vi "Read and Write type1.vi"(8 "error in":errorcluster, 9 "IN":T1(array[cluster]), 10 "Enum":enum16{"Init", "Read", "Write"}(ring), 11 "Path Out":path) -> (0 "error out":errorcluster, 1 "OUT":T1(array[cluster]))   [LabVIEW 2018]
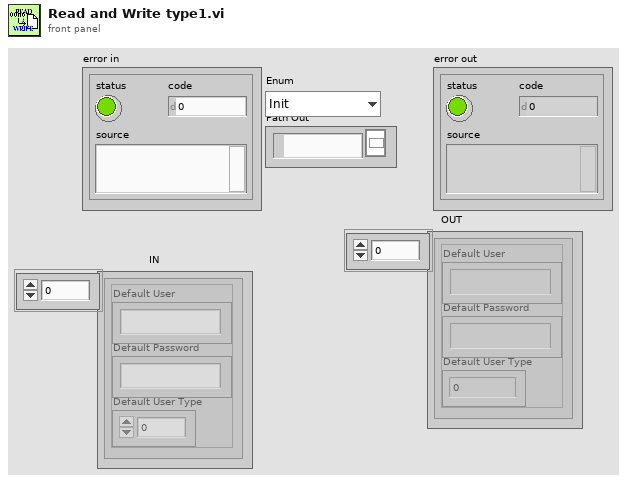
[diagram p1: front panel]
types:
  T1 = cluster{"Default User ":string, "Default Password":string, "Default User Type":u16}[]
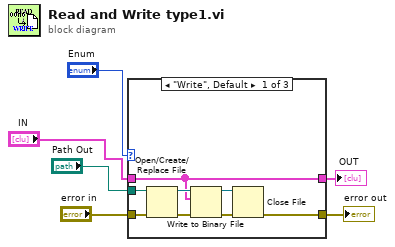
[diagram p0: block diagram]
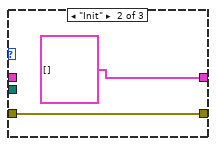
[diagram p2: hidden frame]
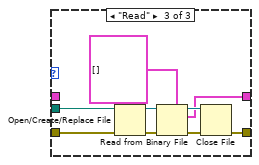
[diagram p3: hidden frame]
diagram:
  n1 = case shown="\"Write\", Default" "Enum" {
    tunnel: "Path Out" -> [w9 _ w21]
    tunnel: "error in" -> [w10 w16 w20]
    tunnel: [w8 w16 w19] -> w4
    tunnel: "IN" -> [w7 _ _]
    tunnel: [w7 T1 [] ("Array") w18] -> w1
    frame "Write", Default {
      n2 = Open/Create/Replace File(file path (use dialog)=w9, error in=w10) -> (refnum out=w11:refnum<file>, error out=w14:errorcluster)  [unwired: 4 in, 1 out]
      n3 = Write to Binary File(file (use dialog)=w11, data=w7, error in=w14) -> (refnum out=w12:refnum<file>, error out=w13:errorcluster)  [unwired: 3 in, 1 out]
      n4 = Close File(refnum=w12, error in=w13) -> (error out=w8:errorcluster)  [unwired: 1 out]
    }
    frame "Init" {
    }
    frame "Read" {
      n5 = Open/Create/Replace File(file path (use dialog)=w21, error in=w20) -> (refnum out=w22:refnum<file>, error out=w25:errorcluster)  [unwired: 4 in, 1 out]
      n6 = Read from Binary File(5:T1 [] ("Array"), 8:w25, 11:w22) -> (0:w24:errorcluster, 2:w18:T1, 3:w23:refnum<file>)  [unwired: 3 in, 1 out]
      n7 = Close File(refnum=w23, error in=w24) -> (error out=w19:errorcluster)  [unwired: 1 out]
    }
  }
  "error out" <- w4
  "OUT" <- w1
